vi "Find and Replace in Text File.vi"(6 "file name":string, 8 "error in":errorcluster, 9 "replace array":string[](array[string]), 10 "find array":string[](array[string]), 11 "folder path":path) -> (0 "error out":errorcluster, 2 "number of replacements":i32[](array[numeric]))   [LabVIEW 2020, in "Template Tool.lvlib"]
uses:
  Template Tool.lvlib
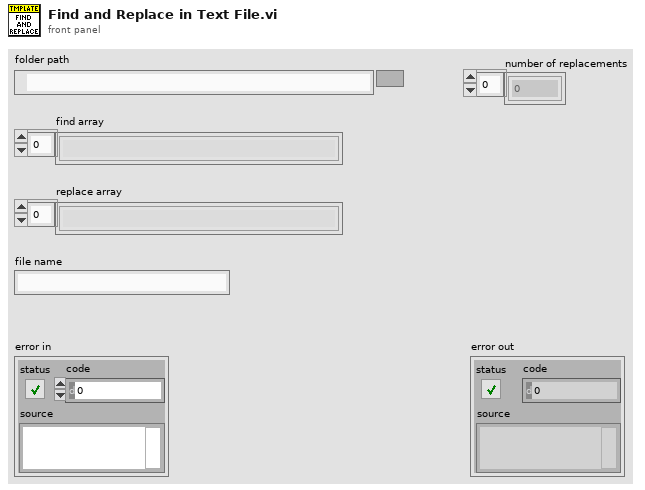
[diagram p1: front panel]
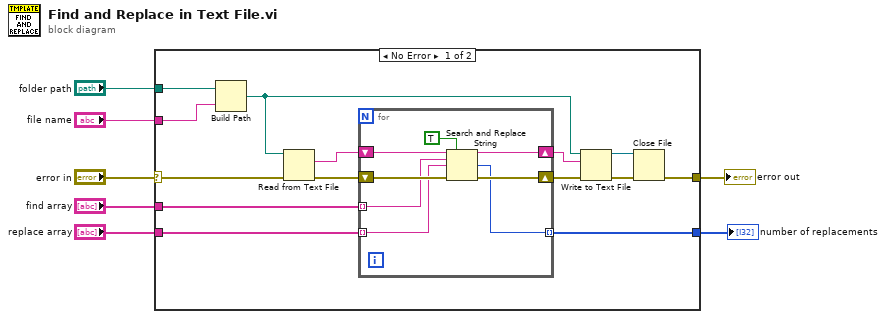
[diagram p0: block diagram]
diagram:
  n1 = case shown="No Error" "error in" {
    selector: "error in" -> [w18 w30]
    tunnel: "folder path" -> [w13 _]
    tunnel: [w15 w30] -> w7
    tunnel: "file name" -> [w8 _]
    tunnel: "find array" -> [w12 _]
    tunnel: "replace array" -> [w11 _]
    tunnel: [w10 _] -> w1
    frame No Error {
      n2 = Build Path(base path=w13, name or relative path=w8) -> (appended path=w21:path)
      n3 = Read from Text File(file (use dialog)=w21, error in=w18) -> (text=w20:string, error out=w9:errorcluster)  [unwired: 2 in, 2 out]
      n4 = for {
        shift-right: [w26] -> w17
        shift-left: w20 -> [w29]
        shift-right: [w25] -> w16
        shift-left: w9 -> [w28]
        tunnel: w12 -> [w24] mode=indexing
        tunnel: w11 -> [w23] mode=indexing
        tunnel: [w22] -> w10 mode=indexing
        n5 = Search and Replace String(replace all?=TRUE ("replace all? (F)"), input string=w29, search string=w24, replace string=w23, error in=w28) -> (result string=w26:string, number of replacements=w22:i32, error out=w25:errorcluster)  [unwired: 3 in, 1 out]
      }
      n6 = Write to Text File(file (use dialog)=w21, text=w17, error in=w16) -> (refnum out=w14:refnum<file>, error out=w19:errorcluster)  [unwired: 1 in, 1 out]
      n7 = Close File(refnum=w14, error in=w19) -> (error out=w15:errorcluster)  [unwired: 1 out]
    }
    frame Error {
    }
  }
  "error out" <- w7
  "number of replacements" <- w1
